vi "Demo v1.vi"() -> ()   [LabVIEW 2013]
panel:
  out "Fail!":bool
  in  "a":dbl=-0.3
  in  "Jump speed":dbl=3.0
  in  "Jump":bool
  out "Picture":i32[][](graph)
  in  "stop":bool
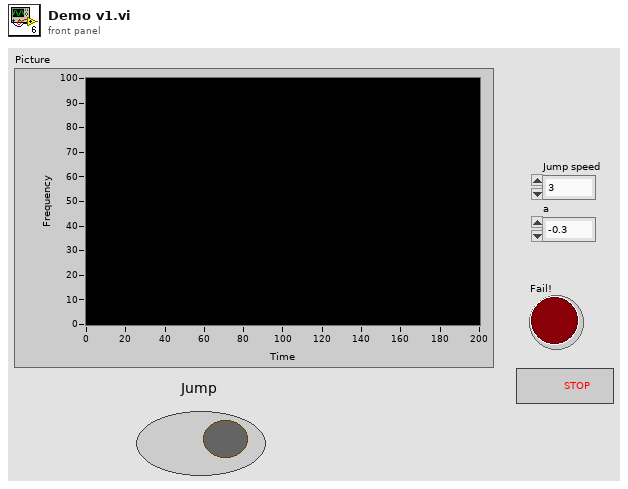
[diagram p1: front panel]
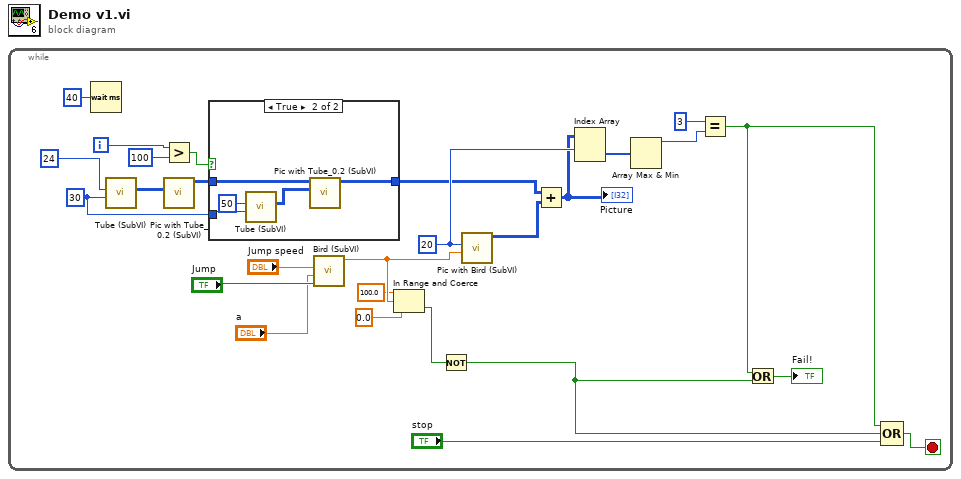
[diagram p0: block diagram]
diagram:
  n1 = while {
    i -> [w18]
    stop <- w14 stop-if-true
    w6 = 20 ("X position")
    w15 = 30 ("Gap height (30)")
    n2 = Wait (ms)(milliseconds to wait=u32 40) -> ()  [unwired: 1 out]
    n3 = call "Tube (SubVI).vi"("Gap height (30)"=w15, "Gap low y"=24) -> ("Tube"=w20:i32[][])  [unwired: 9 in]
    n4 = Greater?(x=w18, y=100) -> (0:w16:bool)
    n5 = call "Pic with Tube_0.2 (SubVI).vi"("Tube"=w20) -> ("Picture"=w19:i32[][])  [unwired: 10 in]
    n6 = case shown="True" w16 {
      tunnel: [w28 w32] -> w5
      tunnel: w19 -> [w28 w33]
      tunnel: w15 -> [_ w30]
      frame False {
      }
      frame True {
        n7 = call "Tube (SubVI).vi"("Gap height (30)"=w30, "Gap low y"=50) -> ("Tube"=w31:i32[][])  [unwired: 9 in]
        n8 = call "Pic with Tube_0.2 (SubVI).vi"("Tube"=w31, "Picture in"=w33) -> ("Picture"=w32:i32[][])  [unwired: 9 in]
      }
    }
    n9 = call "Bird (SubVI).vi"("Jump"="Jump", "a"="a", "Jump speed"="Jump speed") -> ("Position"=w13:dbl)  [unwired: 8 in]
    n10 = In Range and Coerce(upper limit=100.0, x=w13, lower limit=0.0) -> (In Range?=w10:bool)  [unwired: 1 out]
    n11 = Not(x=w10) -> (.not. x?=w3:bool)
    n12 = call "Pic with Bird (SubVI).vi"("Bird Position"=w13, "X position"=w6) -> ("Picture"=w24:i32[][])  [unwired: 9 in]
    n13 = Add(x=w5, y=w24) -> (x+y=w4:i32[][])
    "Picture" <- w4
    n14 = Index Array(array=w4, index (row)=w6) -> (element=w9:i32[])  [unwired: 1 in]
    n15 = Array Max & Min(array=w9) -> (max value=w8:i32)  [unwired: 3 out]
    n16 = Equal?(x=3 ("y"), y=w8) -> (x = y?=w2:bool)
    n17 = Or(x=w2, y=w3) -> (x .or. y?=→"Fail!":bool)
    n18 = Compound Arithmetic op=OR(w2, w3, "stop") -> (w14:bool)
  }
